vi "Create File (full) (N.O.).vi"(8 "error in":errorcluster, 10 "filepath (T)":bool=TRUE, 11 "pathname":path caption="Path Name") -> (0 "error out":errorcluster, 2 "actiontaken?":bool, 3 "pathOUT":path)   [LabVIEW 2015]
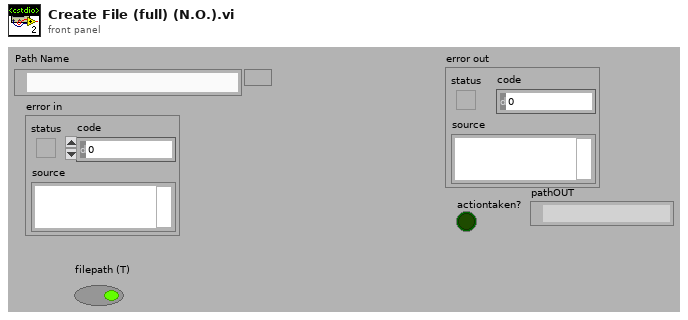
[diagram p1: front panel]
types:
  T1 = enum16{"open", "replace", "create", "open or create", "replace or create", "replace or create with confirmation"}
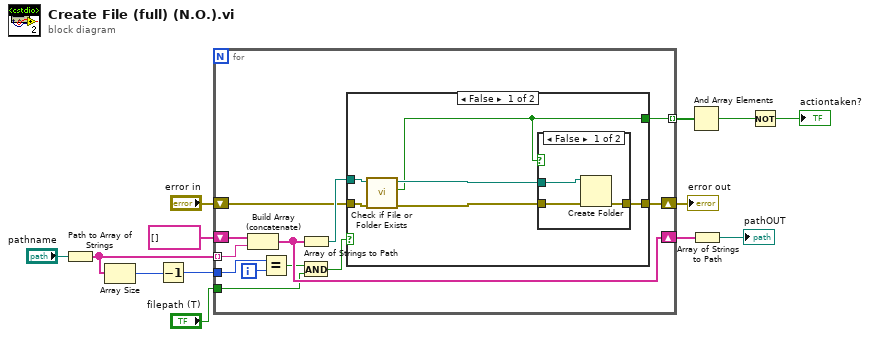
[diagram p0: block diagram]
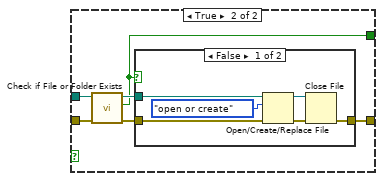
[diagram p3: hidden frame]
diagram:
  n1 = Path to Array of Strings(0:"pathname") -> (2:w11:string[])  [unwired: 1 out]
  n2 = Array Size(array=w11) -> (size(s)=w10:i32)
  n3 = Decrement(x=w10) -> (x-1=w9:i32)
  n4 = for {
    tunnel: w11 -> [w25] mode=indexing
    shift-right: [w23] -> w3
    shift-left: string[] [] -> [w22]
    shift-right: [w20] -> w7
    shift-left: "error in" -> [w21]
    tunnel: w9 -> [w18]
    tunnel: [w17] -> w6 mode=indexing
    tunnel: "filepath (T)" -> [w15]
    i -> [w19]
    n5 = Build Array (concatenate)(w22, w25) -> (w23:string[])
    n6 = Equal?(x=w18, y=w19) -> (x = y?=w16:bool)
    n7 = Array of Strings to Path(0:w23) -> (2:w24:path)  [unwired: 1 in]
    n8 = And(x=w16, y=w15) -> (x .and. y?=w14:bool)
    n9 = case shown="False" w14 {
      tunnel: w24 -> [w31 w41]
      tunnel: w21 -> [w30 w40]
      tunnel: [w28 w38] -> w20
      tunnel: [w26 w36] -> w17
      frame False {
        n10 = call <vilib>:"Check if File or Folder Exists.vi"("error in (no error)"=w30, "path"=w31) -> ("error out"=w29:errorcluster, "file or folder exists?"=w26:bool, "dup path"=w27:path)  [unwired: 7 out]
        n11 = case shown="False" w26 {
          tunnel: w29 -> [w34 w35]
          tunnel: [w33 w35] -> w28
          tunnel: w27 -> [w32 _]
          frame False {
            n12 = Create Folder(path (use dialog)=w32, error in=w34) -> (error out=w33:errorcluster)  [unwired: 3 out]
          }
          frame True {
          }
        }
      }
      frame True {
        n13 = call <vilib>:"Check if File or Folder Exists.vi"("error in (no error)"=w40, "path"=w41) -> ("error out"=w39:errorcluster, "file or folder exists?"=w36:bool, "dup path"=w37:path)  [unwired: 7 out]
        n14 = case shown="False" w36 {
          tunnel: w39 -> [w47 w48]
          tunnel: [w43 w48] -> w38
          tunnel: w37 -> [w46 _]
          frame False {
            n15 = Open/Create/Replace File(file path (use dialog)=w46, error in=w47, operation (0:open)=T1."open or create") -> (refnum out=w44:refnum<file>, error out=w45:errorcluster)  [unwired: 4 out]
            n16 = Close File(refnum=w44, error in=w45) -> (error out=w43:errorcluster)  [unwired: 1 out]
          }
          frame True {
          }
        }
      }
    }
  }
  "error out" <- w7
  n17 = And Array Elements(Boolean array=w6) -> (logical AND=w5:bool)
  n18 = Array of Strings to Path(0:w3) -> (2:→"pathOUT":path)  [unwired: 1 out]
  n19 = Not(x=w5) -> (.not. x?=→"actiontaken?":bool)
